vi "LinFM chirp.vi"() -> ()   [LabVIEW 2019, in "mmW_commands.lvlib"]
uses:
  <vilib>/Analysis/4window.llb/windowTd.ctl
  <vilib>/measure/maspectr.llb/FFT Power Spectrum and PSD for 1 Chan (CDB).vi
  mmW_commands.lvlib
  <vilib>/measure/NI_MAPro.lvlib
  <vilib>/Analysis/NI_AALPro.lvlib
panel:
  in  "Method 1 (T) / Method 2 (F)":bool
  out "Power Spectrum / PSD":cluster{"f0":dbl, "df":dbl, "magnitude":dbl[]}(graph)
  out "Q":dbl[](array[numeric])
  out "I":dbl[](array[numeric])
  in  "span [%]":dbl=80.0
  in  "# of samples":i32=10000
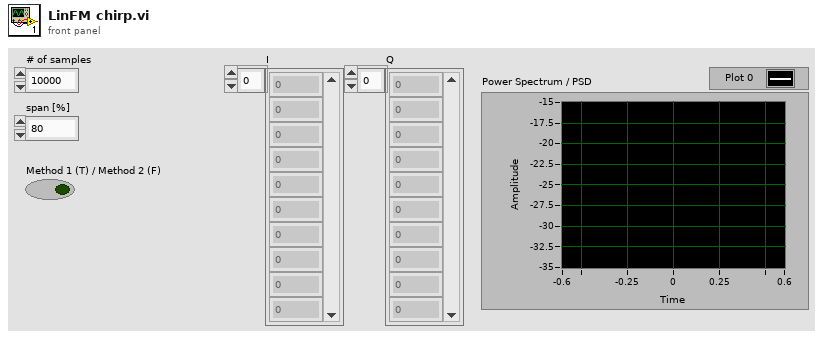
[diagram p1: front panel]
types:
  T1 = typedef "NI_AALPro.lvlib/windowTd.ctl" = u32
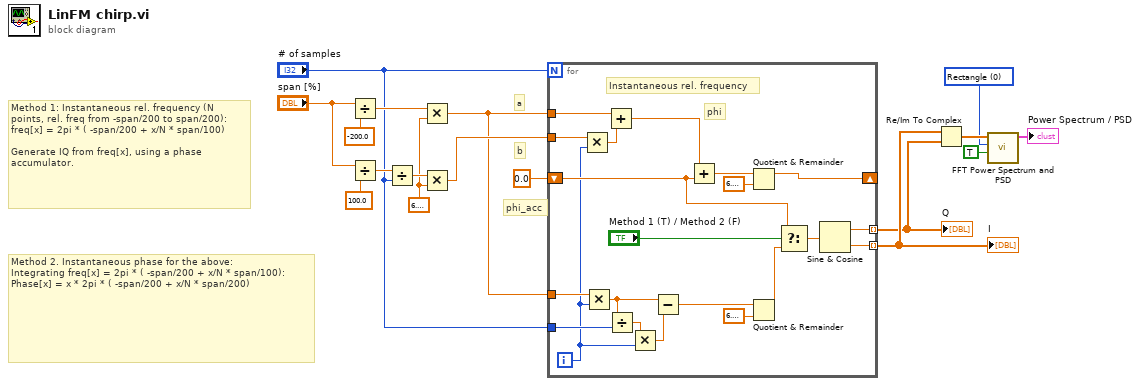
[diagram p0: block diagram]
diagram:
  w2 = T1 0 items=["Rectangle"=0, "Hanning"=1, "Hamming"=2, "Blackman-Harris"=3, "Exact Blackman"=4, "Blackman"=5, "Flat Top"=6, "4 Term B-Harris "=7, "7 Term B-Harris"=8, "Low Sidelobe"=9, "Blackman Nuttall"=11, "Triangle"=30, "Bartlett-Hanning"=31, "Bohman"=32, "Parzen"=33, "Welch"=34, "Kaiser"=60, "Dolph-Chebyshev"=61, "Gaussian"=62] ("window")
  w10 = 6.283185307179586
  # "phi_acc"
  # "b"
  # "a"
  # "Method 2. Instantaneous phase for the above:\nIntegrating freq[x] = 2pi * ( -span/200 + x/N * span/100):\nPhase[x] = x * 2pi * ( -span/200 + x/N * span/200)"
  # "Method 1: Instantaneous rel. frequency (N points, rel. freq from -span/200 to span/200):\nfreq[x] = 2pi * ( -span/200 + x/N * span/100)\n\nGenerate IQ from freq[x], using a phase accumulator."
  n1 = Divide(x="span [%]", y=-200.0) -> (x/y=w15:dbl)
  n2 = Divide(x="span [%]", y=100.0) -> (x/y=w12:dbl)
  n3 = Divide(x=w12, y="# of samples") -> (x/y=w11:dbl)
  n4 = Multiply(x=w15, y=w10) -> (x*y=w8:dbl)
  n5 = Multiply(x=w11, y=w10) -> (x*y=w9:dbl)
  n6 = for {
    N: "# of samples" -> [_]
    tunnel: w8 -> [w34]
    shift-right: [w23] -> _
    shift-left: 0.0 -> [w21]
    tunnel: w9 -> [w36]
    tunnel: [w32] -> w6 mode=indexing
    tunnel: [w31] -> w5 mode=indexing
    tunnel: w8 -> [w30]
    tunnel: "# of samples" -> [w29]
    i -> [w19]
    # "phi"
    # "Instantaneous rel. frequency"
    n7 = Multiply(x=w36, y=w19) -> (x*y=w35:dbl)
    n8 = Multiply(x=w30, y=w19) -> (x*y=w27:dbl)
    n9 = Add(x=w34, y=w35) -> (x+y=w33:dbl)
    n10 = Divide(x=w27, y=w29) -> (x/y=w28:dbl)
    n11 = Multiply(x=w28, y=w19) -> (x*y=w26:dbl)
    n12 = Subtract(x=w27, y=w26) -> (x-y=w25:dbl)
    n13 = Add(x=w33, y=w21) -> (x+y=w37:dbl)
    n14 = Quotient & Remainder(x=w37, y=6.283185307179586) -> (x-y*floor(x/y)=w23:dbl)  [unwired: 1 out]
    n15 = Quotient & Remainder(x=w25, y=6.283185307179586) -> (x-y*floor(x/y)=w20:dbl)  [unwired: 1 out]
    n16 = Select(t=w21, s="Method 1 (T) / Method 2 (F)", f=w20) -> (s? t:f=w22:dbl)
    n17 = Sine & Cosine(0:w22) -> (1:w31:dbl, 2:w32:dbl)
  }
  "I" <- w6
  "Q" <- w5
  n18 = Re/Im To Complex(1:w5, 2:w6) -> (0:w4:cdb[])
  n19 = call-poly <vilib>:"FFT Power Spectrum and PSD.vi"("dB On (F)"=TRUE, "window"=w2, "time signal"=w4) -> ("Power Spectrum / PSD"=→"Power Spectrum / PSD":cluster{"f0":dbl, "df":dbl, "magnitude":dbl[]})  [unwired: 5 in, 3 out]
